vi "listbox1.vi"() -> ()   [LabVIEW 2015]
panel:
  in  "Listbox":i32[](listbox)
  out "Signals":dbl[](graph)
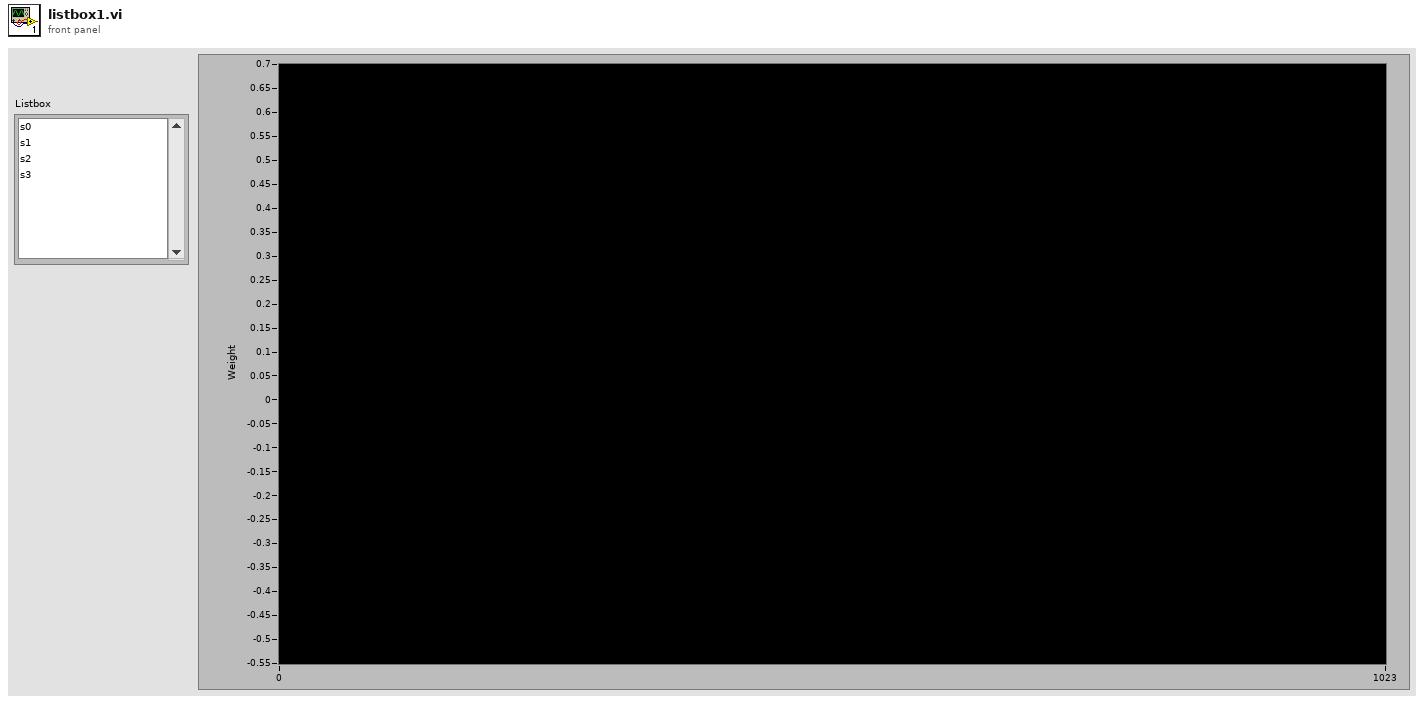
[diagram p1: front panel]
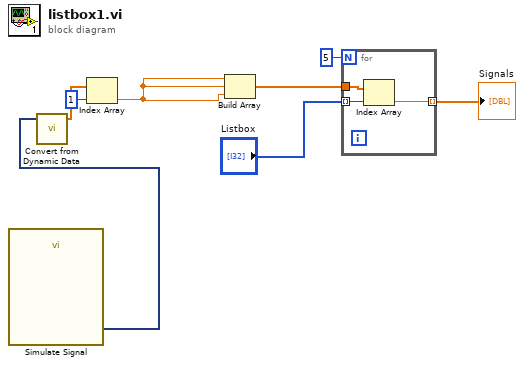
[diagram p0: block diagram]
diagram:
  n1 = call "Simulate Signal"() -> ("Sine with Uniform Noise"=w6:dynamicdata)  [unwired: 14 in, 1 out]
  n2 = call "Convert from Dynamic Data"("Dynamic Data Type"=w6) -> ("Array"=w3:dbl[])  [unwired: 3 in]
  n3 = Index Array(array=w3, index=1) -> (element=w2:dbl)
  n4 = Build Array(w2, w2, w2) -> (w8:dbl[])
  n5 = for {
    N: 5 -> [_]
    tunnel: w8 -> [w11]
    tunnel: "Listbox" -> [w10] mode=indexing
    tunnel: [w9] -> w5 mode=indexing
    n6 = Index Array(array=w11, index=w10) -> (element=w9:dbl)
  }
  "Signals" <- w5
